vi "re_LuaVIEW Do Script.vi"(0 "script file or name (no name)":path, 5 "custom search directory (none)":path, 7 "script string (\"\" == load from file)":string, 11 "error in (no error)":errorcluster) -> (15 "error out":errorcluster)   [LabVIEW 2012]
doc: "Compiles and executes a script while also opening and closing the LuaVIEW reference (which creates and destroys a virtual machine instance) required for this purpose. Use the primitives instead of this VI when manipulation of the script execution state is required."
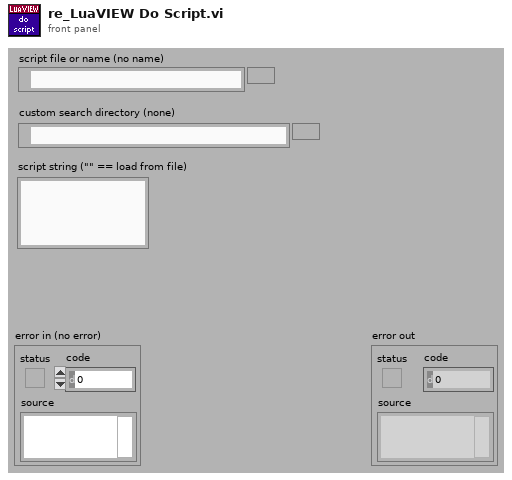
[diagram p1: front panel]
types:
  T1 = typedef "t_LuaVIEW Reference.ctl" = refnum<k1>
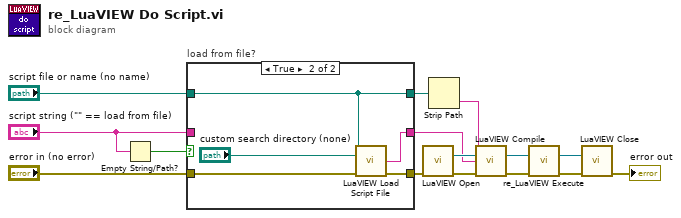
[diagram p0: block diagram]
diagram:
  n1 = Empty String/Path?(string/path="script string (\"\" == load from file)") -> (empty?=w6:bool)
  n2 = case "load from file?" shown="True" w6 {
    tunnel: [w17 w23] -> w8
    tunnel: "error in (no error)" -> [w17 w22]
    tunnel: "script string (\"\" == load from file)" -> [w18 _]
    tunnel: [w18 w20] -> w4
    tunnel: "script file or name (no name)" -> [w16 w19]
    tunnel: [w16 w19] -> w2
    frame False {
    }
    frame True {
      n3 = call "LuaVIEW Load Script File.vi"("script file"=w19, "custom search directory (none)"="custom search directory (none)", "error in (no error)"=w22) -> ("script text"=w20:string, "error out"=w23:errorcluster)  [unwired: 8 in, 3 out]
    }
  }
  n4 = call "LuaVIEW Open.vi"("error in (no error)"=w8) -> ("LuaVIEW reference"=w12:T1, "error out"=w15:errorcluster)  [unwired: 13 in]
  n5 = Strip Path(path=w2) -> (name=w1:string)  [unwired: 1 out]
  n6 = call "LuaVIEW Compile.vi"("script name"=w1, "LuaVIEW reference in"=w12, "script"=w4, "error in (no error)"=w15) -> ("LuaVIEW reference out"=w13:T1, "error out"=w14:errorcluster)  [unwired: 10 in]
  n7 = call "re_LuaVIEW Execute.vi"("LuaVIEW reference in"=w13, "error in (no error)"=w14) -> ("LuaVIEW reference out"=w10:T1, "error out"=w11:errorcluster)  [unwired: 12 in]
  n8 = call "LuaVIEW Close.vi"("LuaVIEW reference"=w10, "error in (no error)"=w11) -> ("dup error"=→"error out":errorcluster)  [unwired: 13 in]
